vi "singleBP.vi"(7 "Expected":dbl, 8 "AccelValue":dbl, 9 "Weight":dbl, 10 "Output":dbl, 11 "LearningFactor":dbl) -> (3 "NewWeight":dbl)   [LabVIEW 2014]
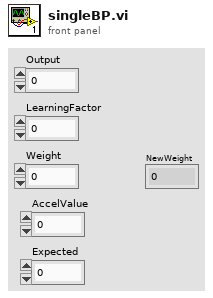
[diagram p1: front panel]
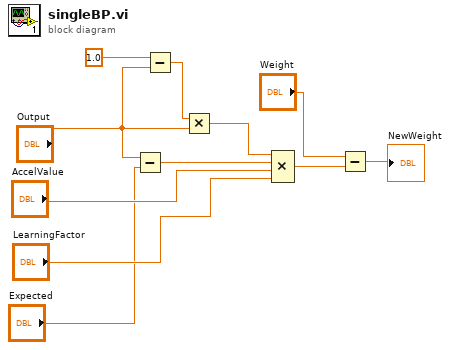
[diagram p0: block diagram]
diagram:
  n1 = Subtract(x="Output", y="Expected") -> (x-y=w11:dbl)
  n2 = Subtract(x=1.0, y="Output") -> (x-y=w9:dbl)
  n3 = Multiply(x=w9, y="Output") -> (x*y=w10:dbl)
  n4 = Compound Arithmetic op=MULTIPLY(w10, w11, "AccelValue", "LearningFactor") -> (w7:dbl)
  n5 = Subtract(x="Weight", y=w7) -> (x-y=→"NewWeight":dbl)
